vi "test Write Data to File.vi"(8 "error in (no error)":errorcluster, 11 "TestCase in":refnum<class "Position Estimation Tests.lvclass">) -> (0 "error out":errorcluster, 3 "TestCase out":refnum<class "Position Estimation Tests.lvclass">)   [LabVIEW 2014, in "Utility VIs tests.lvclass"]
uses:
  Utility VIs tests.lvclass
  Position Estimation Tests/Position Estimation Tests.lvclass
  <vilib>/addons/_JKI Toolkits/VI Tester/TestCase.llb/TestCase.lvclass
  SPLAT/Position.lvclass
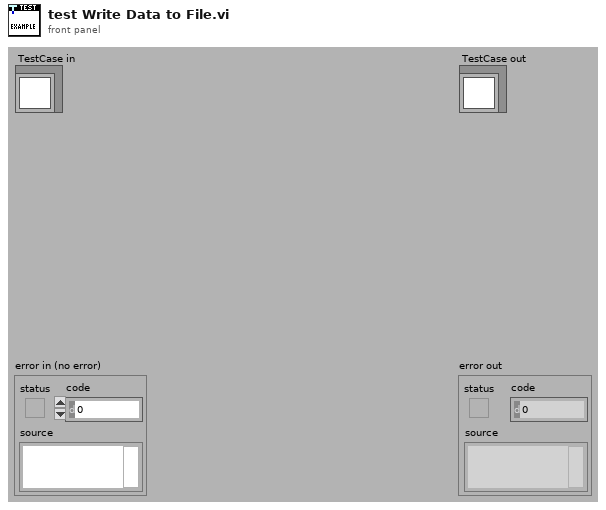
[diagram p1: front panel]
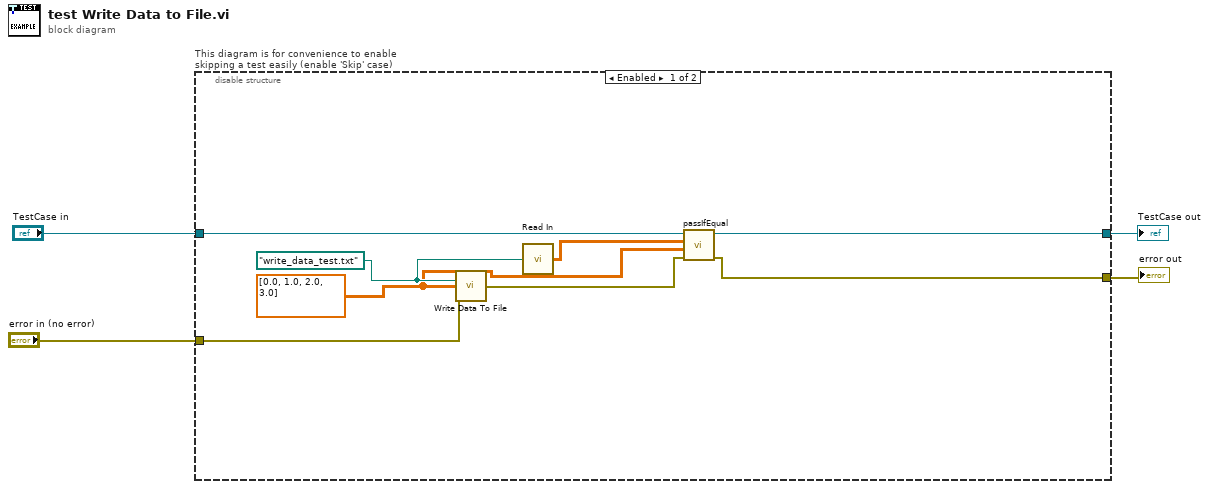
[diagram p0: block diagram]
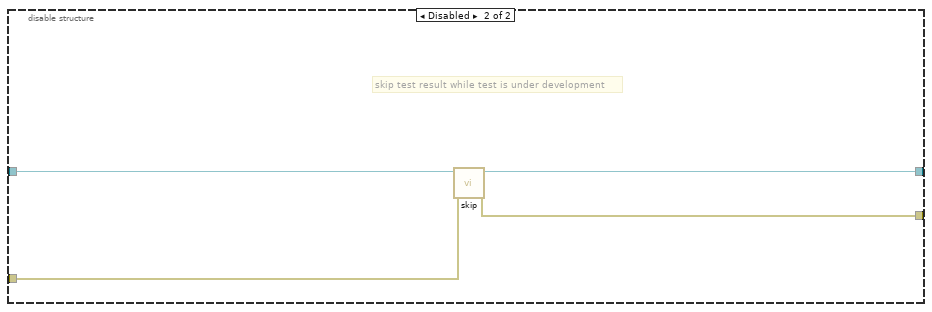
[diagram p2: hidden frame]
diagram:
  n1 = disable-structure "This diagram is for convenience to enable skipping a test easily (enable 'Skip' case)" shown="Enabled" {
    disable-tunnel: "TestCase in" -> [w9 w16]
    disable-tunnel: [w8 w14] -> w1
    disable-tunnel: [w10 w15] -> w3
    disable-tunnel: "error in (no error)" -> [w12 w13]
    frame Enabled {
      w5 = dbl[][] [[0.0, 1.0, 2.0, 3.0]] ("Array")
      w7 = path "write_data_test.txt" ("file path (use dialog)")
      n2 = call "Write Data To File.vi"("file path (use dialog)"=w7, "Array"=w5, "error in"=w12) -> ("error out"=w11:errorcluster)  [unwired: 12 in]
      n3 = call "Read In.vi"("File path"=w7) -> ("DataOut [tagID, anchorID, distance, time]"=w6:dbl[][])  [unwired: 14 in]
      n4 = call-dynamic "passIfEqual.vi"("error in (no error)"=w11, "y"=w5, "x"=w6, "TestCase in"=w9) -> ("error out"=w10:errorcluster, "TestCase out"=w8:refnum<class "Position Estimation Tests.lvclass">)  [unwired: 6 in]
    }
    frame Disabled {
      # "skip test result while test is under development"
      n5 = call <vilib>:"skip.vi"("error in (no error)"=w13, "TestCase in"=w16) -> ("error out"=w15:errorcluster, "TestCase out"=w14:refnum<class "Position Estimation Tests.lvclass">)  [unwired: 8 in]
    }
  }
  "error out" <- w3
  "TestCase out" <- w1
